vi "AH2700_Splitt_Cluster.vi"(0 "AH 2700-Cluster":T3={"Units Display"=1, "Sample Switch"=0, "Frequency"=0.0, "V excitation"=0.0, "Capacity Graphic"=[], "Loss Graphic"=[], "Capacity"=0.0, "Loss"=0.0, "Update AH2500"=FALSE, "Bias "=0.0, " AVerage"=0.0} {"V excitation" format="%#_6f"; "Units Display" items=["nanosiemens"=1, "dissipation factor"=2, "kilohms"=3, "gigohms"=4, "loss vector (jpF)"=5]}) -> (1 "AH2700-Control":T1, 3 "AH 2700-Status":T2={"Units Display"=1, "Sample Switch"=0, "Frequency"=0.0, "V excitation"=0.0, "Capacity Graphic"=[], "Loss Graphic"=[], "Capacity"=0.0, "Loss"=0.0, "Bias "=0.0, " AVerage"=0.0} {"V excitation" format="%#_6f"; "Units Display" items=["nanosiemens"=1, "dissipation factor"=2, "kilohms"=3, "gigohms"=4, "loss vector (jpF)"=5]})   [LabVIEW 2019]
uses:
  AH2700/AH2700-Cluster.ctl
  AH2700/AH2700-Status.ctl
  AH2700/AH2700-Control.ctl
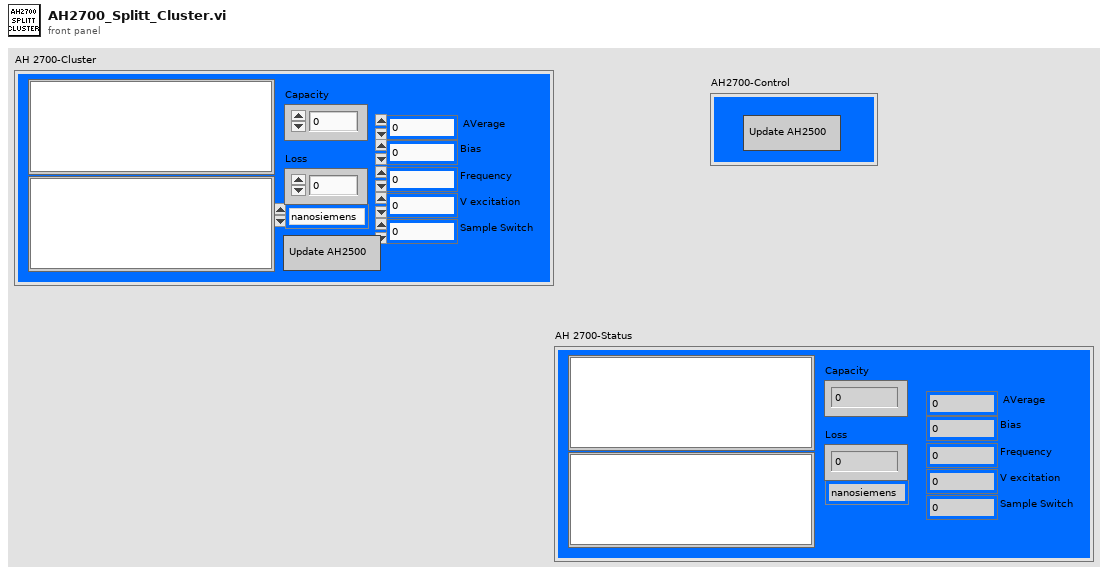
[diagram p1: front panel]
types:
  T1 = typedef "AH2700-Control.ctl" = cluster{"Update AH2500":bool}
  T2 = typedef "AH2700-Status.ctl" = cluster{"Units Display":i32, "Sample Switch":i32, "Frequency":dbl, "V excitation":dbl, "Capacity Graphic":dbl[][], "Loss Graphic":dbl[][], "Capacity":dbl, "Loss":dbl, "Bias ":dbl, " AVerage":dbl}
  T3 = typedef "AH2700-Cluster.ctl" = cluster{"Units Display":i32, "Sample Switch":i32, "Frequency":dbl, "V excitation":dbl, "Capacity Graphic":dbl[][], "Loss Graphic":dbl[][], "Capacity":dbl, "Loss":dbl, "Update AH2500":bool, "Bias ":dbl, " AVerage":dbl}
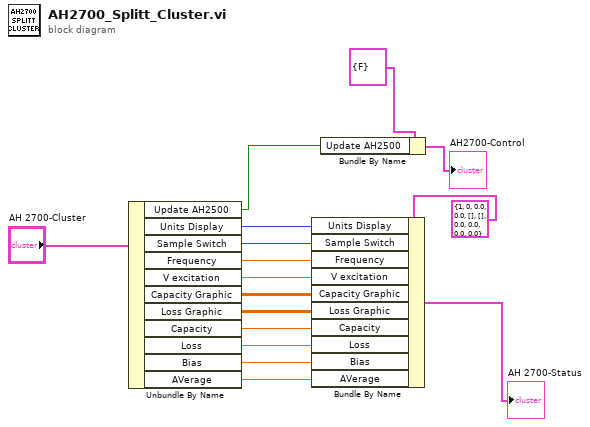
[diagram p0: block diagram]
diagram:
  n1 = Unbundle By Name("AH 2700-Cluster") -> ("Update AH2500"=w11:bool, "Units Display"=w10:i32, "Sample Switch"=w9:i32, "Frequency"=w8:dbl, "V excitation"=w7:dbl, "Capacity Graphic"=w6:dbl[][], "Loss Graphic"=w5:dbl[][], "Capacity"=w4:dbl, "Loss"=w3:dbl, "Bias"=w2:dbl, "AVerage"=w1:dbl)
  n2 = Bundle By Name(cluster=T2 {"Units Display"=1, "Sample Switch"=0, "Frequency"=0.0, "V excitation"=0.0, "Capacity Graphic"=[], "Loss Graphic"=[], "Capacity"=0.0, "Loss"=0.0, "Bias "=0.0, " AVerage"=0.0} ("AH 2700-Status"), "Units Display"=w10, "Sample Switch"=w9, "Frequency"=w8, "V excitation"=w7, "Capacity Graphic"=w6, "Loss Graphic"=w5, "Capacity"=w4, "Loss"=w3, "Bias"=w2, "AVerage"=w1) -> (→"AH 2700-Status":T2)
  n3 = Bundle By Name(cluster=T1 {"Update AH2500"=FALSE} ("AH2700-Control"), "Update AH2500"=w11) -> (→"AH2700-Control":T1)
